vi "Before File Logging.vi"(7 "Configuration":T1={"Delimiter"=",", "Enable Calendar Tree"=FALSE, "File Extension"="csv", "Maximum File Count"=1, "Maximum File Size"=15728640, "Prune All"=FALSE, "Root Folder"=path ""}, 8 "Error In":errorcluster) -> (0 "Error Out":errorcluster, 3 "Test Log Folder":path=path "C:/Users/cfield/AppData/Local/Temp/lvtemporary_667516.tmp")   [LabVIEW 2018, in "Tests.lvlib"]
uses:
  Tests.lvlib
  src/Toolkit/Type Definitions/Configuration.ctl
  src/Toolkit/Toolkit.lvlib
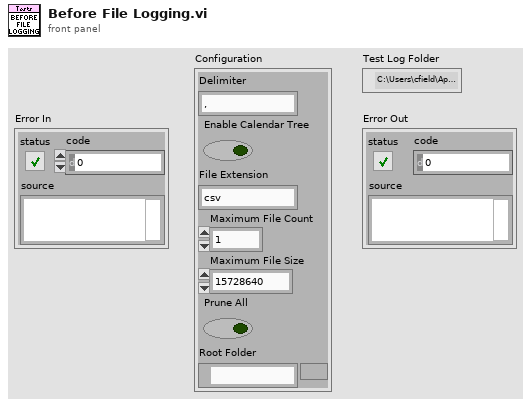
[diagram p1: front panel]
types:
  T1 = typedef "Toolkit.lvlib/Configuration.ctl" = cluster{"Delimiter":string, "Enable Calendar Tree":bool, "File Extension":string, "Maximum File Count":i32, "Maximum File Size":i64, "Prune All":bool, "Root Folder":path}
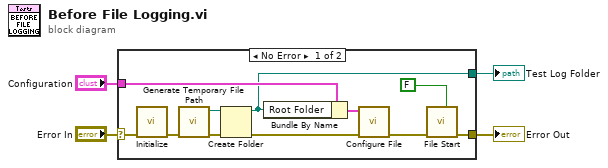
[diagram p0: block diagram]
diagram:
  n1 = case shown="No Error" "Error In" {
    selector: "Error In" -> [w6 w16]
    tunnel: [w15 w16] -> w4
    tunnel: [w10 _] -> w3
    tunnel: "Configuration" -> [w11 _]
    frame No Error {
      n2 = call "Initialize.vi"("Error In"=w6) -> ("Error Out"=w5:errorcluster)  [unwired: 10 in]
      n3 = call <vilib>:"Generate Temporary File Path.vi"("error in (no error)"=w5) -> ("error out"=w14:errorcluster, "Unique Temporary File Path"=w13:path)  [unwired: 9 in]
      n4 = Create Folder(path (use dialog)=w13, error in=w14) -> (created path=w10:path, error out=w8:errorcluster)  [unwired: 1 in, 1 out]
      n5 = Bundle By Name(cluster=w11, "Root Folder"=w10) -> (w9:T1)
      n6 = call "Configure File.vi"("Error In"=w8, "Configuration"=w9) -> ("Error Out"=w7:errorcluster)  [unwired: 9 in]
      n7 = call "File Start.vi"("Run in Background"=FALSE, "Error In"=w7) -> ("Error Out"=w15:errorcluster)  [unwired: 9 in]
    }
    frame Error {
    }
  }
  "Error Out" <- w4
  "Test Log Folder" <- w3
